vi "仪器参数发送 (子VI).vi"(8 "错误输入":errorcluster caption="错误输出") -> (0 "错误输出":errorcluster)   [LabVIEW 2016]
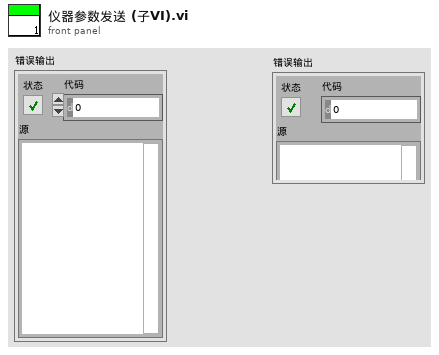
[diagram p1: front panel]
types:
  T1 = cluster{"氨氮仪器参数索引起始时间":string, "总磷仪器参数索引起始时间":string, "总氮仪器参数索引起始时间":string, "CODMn仪器参数索引起始时间":string, "CODCr仪器参数索引起始时间":string, "DO仪器参数索引起始时间":string, "PH仪器参数索引起始时间":string, "比电导率仪器参数索引起始时间":string, "水温仪器参数索引起始时间":string, "浊度仪器参数索引起始时间":string, "叶绿素a仪器参数索引起始时间":string, "藻密度仪器参数索引起始时间":string, "ORP仪器参数索引起始时间":string}
  T2 = cluster{"[0]":string, "[1]":string, "[2]":string, "[3]":string, "[4]":string, "[5]":string, "[6]":string, "[7]":string, "[8]":string, "[9]":string, "[10]":string, "[11]":string, "[12]":string}
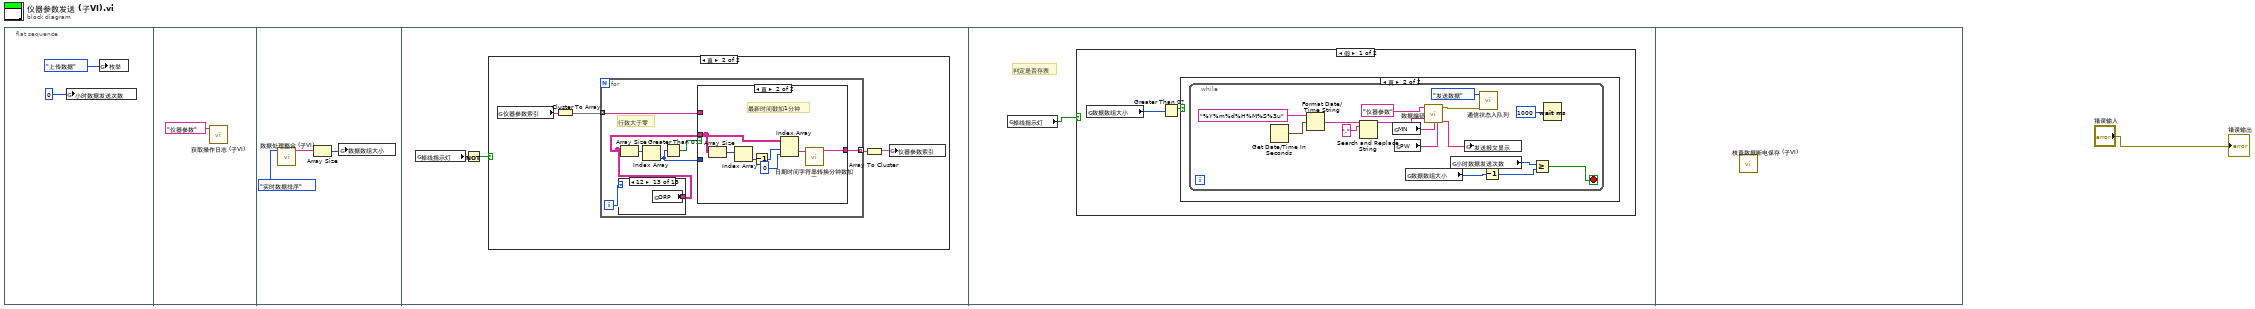
[diagram p0: block diagram]
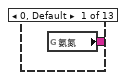
[diagram p3: hidden frame]
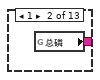
[diagram p4: hidden frame]
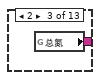
[diagram p5: hidden frame]
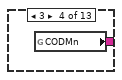
[diagram p6: hidden frame]
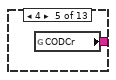
[diagram p7: hidden frame]
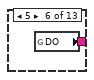
[diagram p8: hidden frame]
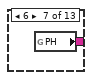
[diagram p9: hidden frame]
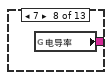
[diagram p10: hidden frame]
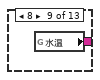
[diagram p11: hidden frame]
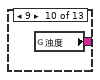
[diagram p12: hidden frame]
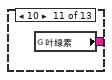
[diagram p13: hidden frame]
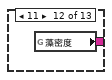
[diagram p14: hidden frame]
diagram:
  n1 = flat-sequence {
    frame #0 {
      n2 = global write "全局 小时数据发送次数.vi" "小时数据发送次数"(0 ("小时数据发送次数")) -> ()
      n3 = global write "全局1.vi" "枚举"(enum16{"返回请求应答", "上传数据", "返回执行结果"}."上传数据" ("枚举")) -> ()
    }
    frame #1 {
      n4 = call "获取操作日志 (子VI).vi"("table输入"="仪器参数") -> ()  [unwired: 11 in]
    }
    frame #2 {
      n5 = call "数据处理整合 (子VI).vi"("枚举"=enum16{"实时数据排序", "小时数据排序"}."实时数据排序") -> ("已排序的数组"=w7:string[])  [unwired: 10 in]
      n6 = Array Size(array=w7) -> (size(s)=w6:i32)
      n7 = global write "全局 数据数组大小.vi" "数据数组大小"(w6) -> ()
    }
    frame #3 {
      n8 = global read "全局 数据发送重叠.vi" "掉线指示灯"() -> (w9:bool)
      n9 = Not(x=w9) -> (.not. x?=w8:bool)
      n10 = case shown="真" w8 {
        frame False {
        }
        frame True {
          n11 = global read "全局 时间2.vi" "仪器参数索引"() -> (w13:T1)
          n12 = Cluster To Array(cluster=w13) -> (array=w12:string[])
          n13 = for {
            tunnel: [w17] -> w10 mode=indexing
            tunnel: w12 -> [w16] mode=indexing
            i -> [w15]
            # "行数大于零"
            n14 = case shown="12" w15 {
              tunnel: [w21 w22 w23 w24 w25 w26 w27 w28 w29 w30 w31 w32 w33] -> w14
              frame 0, Default {
                n15 = global read "全局 所有参数.vi" "氨氮"() -> (w21:string[][])
              }
              frame 1 {
                n16 = global read "全局 所有参数.vi" "总磷"() -> (w22:string[][])
              }
              frame 2 {
                n17 = global read "全局 所有参数.vi" "总氮"() -> (w23:string[][])
              }
              frame 3 {
                n18 = global read "全局 所有参数.vi" "CODMn"() -> (w24:string[][])
              }
              frame 4 {
                n19 = global read "全局 所有参数.vi" "CODCr"() -> (w25:string[][])
              }
              frame 5 {
                n20 = global read "全局 所有参数.vi" "DO"() -> (w26:string[][])
              }
              frame 6 {
                n21 = global read "全局 所有参数.vi" "PH"() -> (w27:string[][])
              }
              frame 7 {
                n22 = global read "全局 所有参数.vi" "电导率"() -> (w28:string[][])
              }
              frame 8 {
                n23 = global read "全局 所有参数.vi" "水温"() -> (w29:string[][])
              }
              frame 9 {
                n24 = global read "全局 所有参数.vi" "浊度"() -> (w30:string[][])
              }
              frame 10 {
                n25 = global read "全局 所有参数.vi" "叶绿素"() -> (w31:string[][])
              }
              frame 11 {
                n26 = global read "全局 所有参数.vi" "藻密度"() -> (w32:string[][])
              }
              frame 12 {
                n27 = global read "全局 所有参数.vi" "ORP"() -> (w33:string[][])
              }
            }
            n28 = Array Size(array=w14) -> (size(s)=w19:i32[])
            n29 = Index Array(array=w19) -> (element=w18:i32)  [unwired: 1 in]
            n30 = Greater Than 0?(x=w18) -> (x > 0?=w20:bool)
            n31 = case shown="真" w20 {
              tunnel: w18 -> [_ _]
              tunnel: w14 -> [_ w38]
              tunnel: [w34 w35] -> w17
              tunnel: w16 -> [w34 _]
              frame False {
              }
              frame True {
                # "最新时间戳加1分钟"
                n32 = Array Size(array=w38) -> (size(s)=w40:i32[])
                n33 = Index Array(array=w40) -> (element=w39:i32)  [unwired: 1 in]
                n34 = Decrement(x=w39) -> (x-1=w37:i32)
                n35 = Index Array(array=w38, index (row)=w37, index (col)=0 ("禁用的索引 (列)")) -> (element=w41:string)
                n36 = call "日期时间字符串转换分钟数加一.vi"("data[0]"=w41) -> ("日期/时间字符串"=w35:string)  [unwired: 10 in]
              }
            }
          }
          n37 = Array To Cluster(array=w10) -> (cluster=w11:T2)
          n38 = global write "全局 时间2.vi" "仪器参数索引"(w11) -> ()
        }
      }
    }
    frame #4 {
      # "判定是否存表"
      n39 = global read "全局 数据发送重叠.vi" "掉线指示灯"() -> (w42:bool)
      n40 = case shown="假" w42 {
        frame False {
          n41 = global read "全局 数据数组大小.vi" "数据数组大小"() -> (w43:i32)
          n42 = Greater Than 0?(x=w43) -> (x > 0?=w44:bool)
          n43 = case shown="真" w44 {
            frame False {
            }
            frame True {
              n44 = while {
                stop <- w45 stop-if-true
                n45 = Get Date/Time In Seconds() -> (seconds since 1Jan1904=w58:timestamp)
                n46 = Format Date/Time String(time format string (%c)="%Y%m%d%H%M%S%3u" ("时间格式字符串(%c)"), seconds (now)=w58) -> (date/time string=w57:string)  [unwired: 1 in]
                n47 = Search and Replace String(input string=w57, search string="." ("搜索字符串")) -> (result string=w55:string)  [unwired: 6 in, 3 out]
                n48 = global read "断电保存全局.vi" "MN"() -> (w52:string)
                n49 = global read "断电保存全局.vi" "PW"() -> (w51:string)
                n50 = global read "全局 数据数组大小.vi" "数据数组大小"() -> (w47:i32)
                n51 = call "数据编码.vi"("table输入"="仪器参数" ("新元素/子数组"), "QN"=w55, "MN"=w52, "PW"=w51) -> ("错误常量"=w50:errorcluster, "通讯包字符串"=w54:string)  [unwired: 10 in]
                n52 = global read "全局 小时数据发送次数.vi" "小时数据发送次数"() -> (w48:i32)
                n53 = global write "全局1.vi" "发送报文显示"(w54) -> ()
                n54 = call "通信状态入队列.vi"("错误输入（无错误）"=w50, "枚举"=enum16{"打开连接", "发送数据", "读取数据", "数据处理", "关闭连接"}."发送数据") -> ()  [unwired: 9 in, 1 out]
                n55 = Decrement(x=w47) -> (x-1=w46:i32)
                n56 = Greater Or Equal?(x=w48, y=w46) -> (x >= y?=w45:bool)
                n57 = Wait (ms)(milliseconds to wait=u32 1000 ("等待时间（毫秒）")) -> ()  [unwired: 1 out]
              }
            }
          }
        }
        frame True {
        }
      }
    }
    frame #5 {
      n58 = call "核查数据断电保存 (子VI).vi"() -> ()  [unwired: 12 in]
    }
  }
  "错误输出" <- "错误输入"
